vi "GetPhaseABCProperties.vi"(8 "error in (no error)":errorcluster, 9 "Channels":T1[](array[typedef]), 10 "Channel Properties":T2[](array[typedef]), 11 "ChannelType":string) -> (0 "error out":errorcluster, 2 "AssetIdABC":string[](array[string]), 3 "AssetNameABC":string[](array[string]))   [LabVIEW 2017, in "McsaTestPanel.lvlib"]
uses:
  <vilib>/addons/InsightCM/Devices/Shared/Mcsa/McsaTestPanel/McsaTestPanel.lvlib
  <vilib>/addons/InsightCM/MessageBus/Base/controls/KeyValuePair.ctl
  <vilib>/addons/InsightCM/MessageBus/Base/controls/R2_Channel.ctl
  <vilib>/addons/InsightCM/MessageBus/Base/controls/Metric.ctl
  <vilib>/addons/InsightCM/Utilities/PropertyHelpers/PropertyHelpers.lvlib
  <vilib>/addons/InsightCM/Utilities/MCSA/McsaUtilities.lvlib
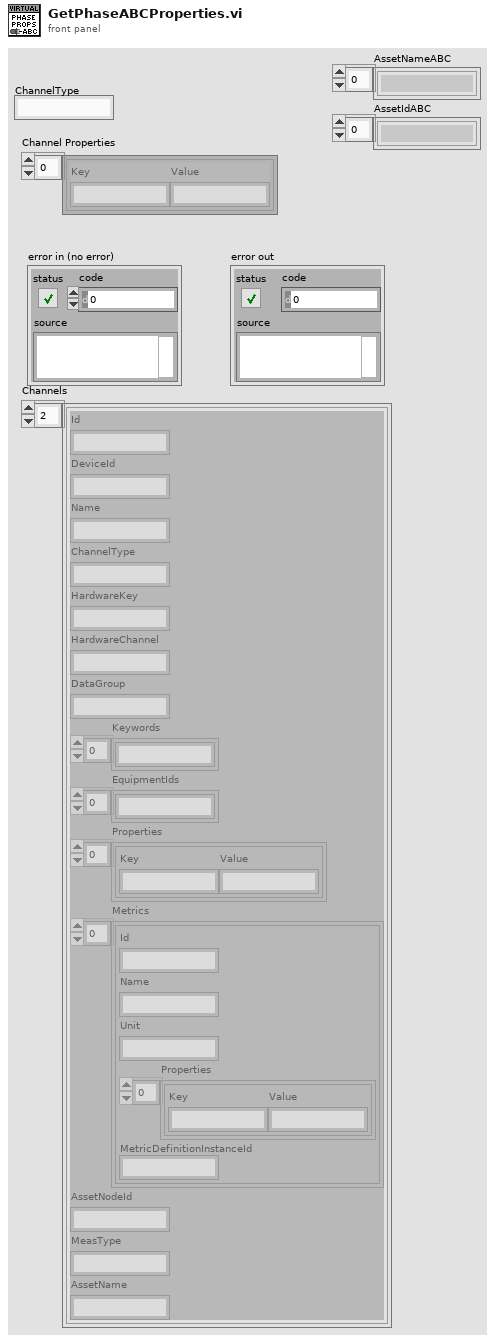
[diagram p1: front panel]
types:
  T1 = typedef "R2_Channel.ctl" = cluster{"Id":string, "DeviceId":string, "Name":string, "ChannelType":string, "HardwareKey":string, "HardwareChannel":string, "DataGroup":string, "Keywords":string[], "EquipmentIds":string[], "Properties":T2[], "Metrics":T3[], "AssetNodeId":string, "MeasType":string, "AssetName":string}
  T2 = typedef "KeyValuePair.ctl" = cluster{"Key":string, "Value":string}
  T3 = typedef "Metric.ctl" = cluster{"Id":string, "Name":string, "Unit":string, "Properties":T2[], "MetricDefinitionInstanceId":string}
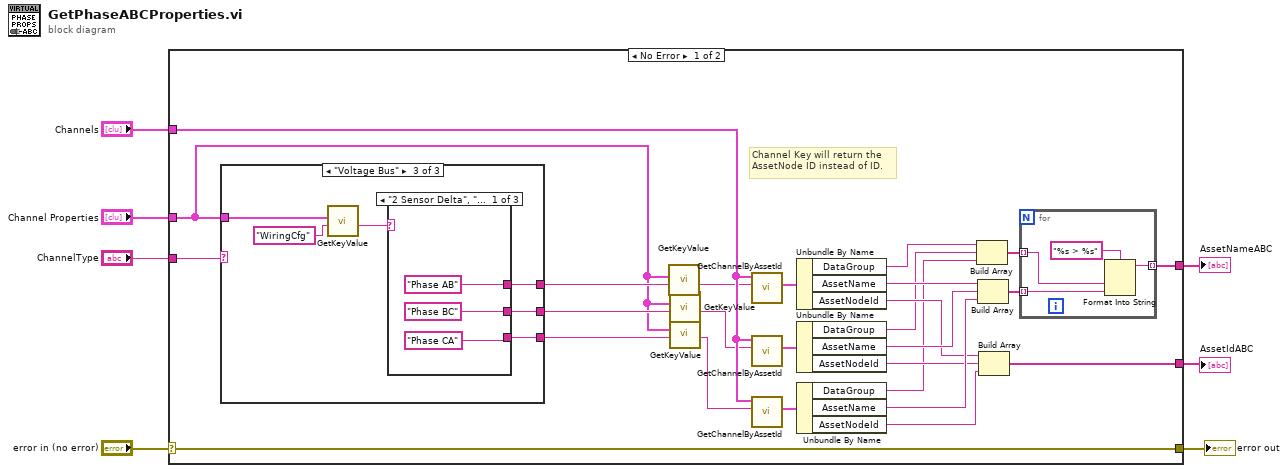
[diagram p0: block diagram]
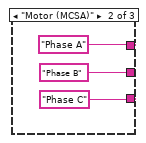
[diagram p3: hidden frame]
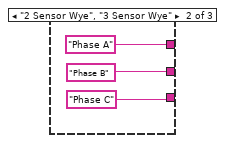
[diagram p4: hidden frame]
diagram:
  n1 = case shown="No Error" "error in (no error)" {
    selector: "error in (no error)" -> [w21 w53]
    tunnel: "ChannelType" -> [w32 _]
    tunnel: "Channels" -> [w29 _]
    tunnel: "Channel Properties" -> [w23 _]
    tunnel: [w21 w53] -> w3
    tunnel: [w12 _] -> w2
    tunnel: [w14 _] -> w1
    frame No Error {
      # "Channel Key will return the\nAssetNode ID instead of ID."
      n2 = case shown="\"Voltage Bus\"" w32 {
        tunnel: w23 -> [_ _ w45]
        tunnel: [_ "Phase C" ("Name") w44] -> w24
        tunnel: [_ "Phase B" ("Name") w43] -> w26
        tunnel: [_ "Phase A" ("Name") w42] -> w28
        frame Default {
        }
        frame "Motor (MCSA)" {
        }
        frame "Voltage Bus" {
          n3 = call <vilib>:"GetKeyValue.vi"("key"="WiringCfg" ("Name"), "key value pairs"=w45) -> ("value"=w41:string)  [unwired: 7 in, 2 out]
          n4 = case shown="\"2 Sensor Delta\", \"3 Sensor Delta\"" w41 {
            tunnel: ["Phase AB" ("Name") "Phase A" ("Name") _] -> w42
            tunnel: ["Phase BC" ("Name") "Phase B" ("Name") _] -> w43
            tunnel: ["Phase CA" ("Name") "Phase C" ("Name") _] -> w44
            frame "2 Sensor Delta", "3 Sensor Delta" {
            }
            frame "2 Sensor Wye", "3 Sensor Wye" {
            }
            frame Default {
            }
          }
        }
      }
      n5 = call <vilib>:"GetKeyValue.vi"("key"=w28, "key value pairs"=w23) -> ("value"=w27:string)  [unwired: 7 in, 2 out]
      n6 = call <vilib>:"GetKeyValue.vi"("key"=w26, "key value pairs"=w23) -> ("value"=w25:string)  [unwired: 7 in, 2 out]
      n7 = call <vilib>:"GetKeyValue.vi"("key"=w24, "key value pairs"=w23) -> ("value"=w22:string)  [unwired: 7 in, 2 out]
      n8 = call <vilib>:"GetChannelByAssetId.vi"("node id"=w27, "channels in"=w29) -> ("channel"=w33:T1)  [unwired: 7 in, 2 out]
      n9 = call <vilib>:"GetChannelByAssetId.vi"("node id"=w25, "channels in"=w29) -> ("channel"=w31:T1)  [unwired: 7 in, 2 out]
      n10 = call <vilib>:"GetChannelByAssetId.vi"("node id"=w22, "channels in"=w29) -> ("channel"=w30:T1)  [unwired: 7 in, 2 out]
      n11 = Unbundle By Name(w33) -> ("DataGroup"=w11:string, "AssetName"=w20:string, "AssetNodeId"=w17:string)
      n12 = Unbundle By Name(w31) -> ("DataGroup"=w9:string, "AssetName"=w19:string, "AssetNodeId"=w16:string)
      n13 = Unbundle By Name(w30) -> ("DataGroup"=w10:string, "AssetName"=w18:string, "AssetNodeId"=w15:string)
      n14 = Build Array(w11, w9, w10) -> (w8:string[])
      n15 = Build Array(w20, w19, w18) -> (w13:string[])
      n16 = Build Array(w17, w16, w15) -> (w14:string[])
      n17 = for {
        tunnel: w13 -> [w35] mode=indexing
        tunnel: [w36] -> w12 mode=indexing
        tunnel: w8 -> [w34] mode=indexing
        n18 = Format Into String(format string="%s > %s", w34, w35) -> (resulting string=w36:string)  [unwired: 2 in, 1 out]
      }
    }
    frame Error {
    }
  }
  "error out" <- w3
  "AssetNameABC" <- w2
  "AssetIdABC" <- w1
